vi "A12rowmm.vi"(11 "Basic Size":dbl) -> (3 "Row":dbl)   [LabVIEW 2023]
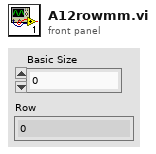
[diagram p1: front panel]
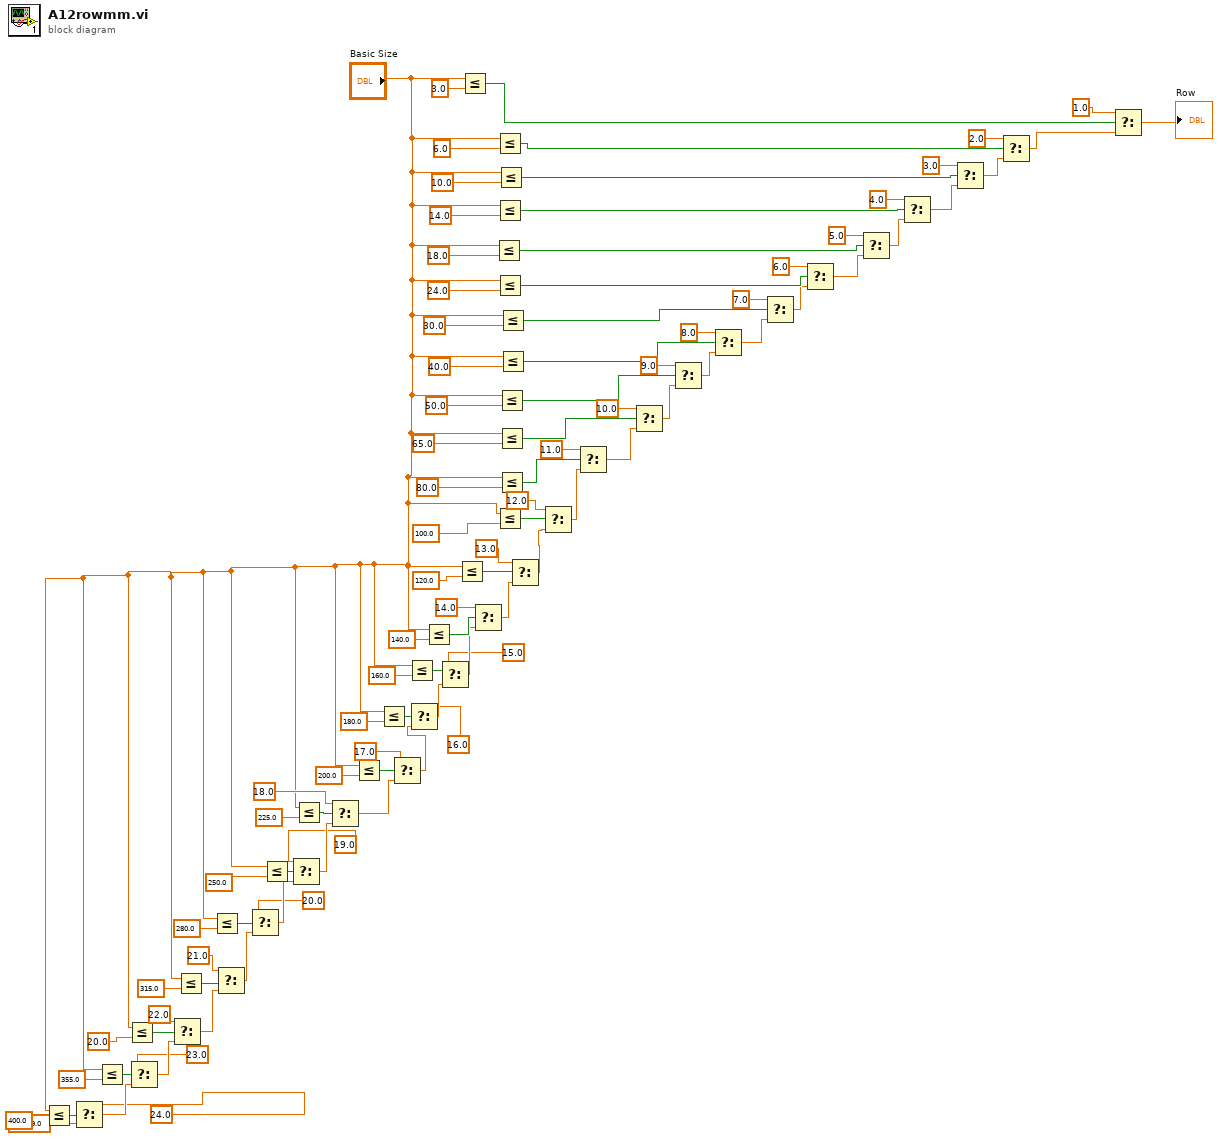
[diagram p0: block diagram]
diagram:
  n1 = Less Or Equal?(x="Basic Size", y=400.0) -> (x <= y?=w6:bool)
  n2 = Select(t=24.0, s=w6, f=999999.0) -> (s? t:f=w8:dbl)
  n3 = Less Or Equal?(x="Basic Size", y=355.0) -> (x <= y?=w11:bool)
  n4 = Less Or Equal?(x="Basic Size", y=20.0 ("t")) -> (x <= y?=w15:bool)
  n5 = Select(t=23.0, s=w11, f=w8) -> (s? t:f=w12:dbl)
  n6 = Select(t=22.0, s=w15, f=w12) -> (s? t:f=w16:dbl)
  n7 = Less Or Equal?(x="Basic Size", y=315.0) -> (x <= y?=w19:bool)
  n8 = Less Or Equal?(x="Basic Size", y=280.0) -> (x <= y?=w23:bool)
  n9 = Select(t=21.0, s=w19, f=w16) -> (s? t:f=w20:dbl)
  n10 = Select(t=20.0, s=w23, f=w20) -> (s? t:f=w24:dbl)
  n11 = Less Or Equal?(x="Basic Size", y=250.0) -> (x <= y?=w27:bool)
  n12 = Select(t=19.0, s=w27, f=w24) -> (s? t:f=w28:dbl)
  n13 = Less Or Equal?(x="Basic Size", y=225.0) -> (x <= y?=w31:bool)
  n14 = Select(t=18.0, s=w31, f=w28) -> (s? t:f=w32:dbl)
  n15 = Less Or Equal?(x="Basic Size", y=200.0) -> (x <= y?=w34:bool)
  n16 = Less Or Equal?(x="Basic Size", y=180.0) -> (x <= y?=w37:bool)
  n17 = Select(t=17.0, s=w34, f=w32) -> (s? t:f=w35:dbl)
  n18 = Less Or Equal?(x="Basic Size", y=160.0) -> (x <= y?=w41:bool)
  n19 = Select(t=16.0, s=w37, f=w35) -> (s? t:f=w38:dbl)
  n20 = Less Or Equal?(x="Basic Size", y=140.0) -> (x <= y?=w44:bool)
  n21 = Select(t=15.0, s=w41, f=w38) -> (s? t:f=w42:dbl)
  n22 = Less Or Equal?(x="Basic Size", y=120.0) -> (x <= y?=w50:bool)
  n23 = Less Or Equal?(x="Basic Size", y=3.0) -> (x <= y?=w97:bool)
  n24 = Select(t=14.0, s=w44, f=w42) -> (s? t:f=w46:dbl)
  n25 = Less Or Equal?(x="Basic Size", y=18.0) -> (x <= y?=w81:bool)
  n26 = Less Or Equal?(x="Basic Size", y=6.0) -> (x <= y?=w93:bool)
  n27 = Less Or Equal?(x="Basic Size", y=14.0) -> (x <= y?=w85:bool)
  n28 = Less Or Equal?(x="Basic Size", y=24.0) -> (x <= y?=w77:bool)
  n29 = Less Or Equal?(x="Basic Size", y=100.0 ("x")) -> (x <= y?=w55:bool)
  n30 = Less Or Equal?(x="Basic Size", y=10.0) -> (x <= y?=w90:bool)
  n31 = Less Or Equal?(x="Basic Size", y=50.0) -> (x <= y?=w65:bool)
  n32 = Less Or Equal?(x="Basic Size", y=65.0) -> (x <= y?=w61:bool)
  n33 = Less Or Equal?(x="Basic Size", y=80.0) -> (x <= y?=w57:bool)
  n34 = Less Or Equal?(x="Basic Size", y=30.0) -> (x <= y?=w73:bool)
  n35 = Less Or Equal?(x="Basic Size", y=40.0) -> (x <= y?=w69:bool)
  n36 = Select(t=13.0, s=w50, f=w46) -> (s? t:f=w49:dbl)
  n37 = Select(t=12.0, s=w55, f=w49) -> (s? t:f=w54:dbl)
  n38 = Select(t=11.0, s=w57, f=w54) -> (s? t:f=w59:dbl)
  n39 = Select(t=10.0, s=w61, f=w59) -> (s? t:f=w64:dbl)
  n40 = Select(t=9.0, s=w65, f=w64) -> (s? t:f=w67:dbl)
  n41 = Select(t=8.0, s=w69, f=w67) -> (s? t:f=w71:dbl)
  n42 = Select(t=7.0, s=w73, f=w71) -> (s? t:f=w75:dbl)
  n43 = Select(t=6.0, s=w77, f=w75) -> (s? t:f=w79:dbl)
  n44 = Select(t=5.0, s=w81, f=w79) -> (s? t:f=w83:dbl)
  n45 = Select(t=4.0, s=w85, f=w83) -> (s? t:f=w87:dbl)
  n46 = Select(t=3.0, s=w90, f=w87) -> (s? t:f=w91:dbl)
  n47 = Select(t=2.0, s=w93, f=w91) -> (s? t:f=w94:dbl)
  n48 = Select(t=1.0, s=w97, f=w94) -> (s? t:f=→"Row":dbl)
